vi "inverse_transform.vi"(8 "error in (no error)":errorcluster caption="entrée d'erreur (pas d'erreur)", 11 "KernelPCA.lvclass 2":refnum<class "KernelPCA.lvclass">) -> (0 "error out":errorcluster caption="sortie d'erreur", 2 "X":dbl[][](array[numeric]), 3 "KernelPCA.lvclass":refnum<class "KernelPCA.lvclass">)   [LabVIEW 2020, in "KernelPCA.lvclass"]
doc: "Transform X back to original space.\n\n ``inverse_transform`` approximates the inverse transformation using\n a learned pre-image. The pre-image is learned by kernel ridge\n regression of the original data on their low-dimensional representation\n vectors.\n\n .. note:\n :meth:`~sklearn.decomposition.fit` internally uses a centered\n kernel. As the centered kernel no longer contains the information\n of the mean of kernel features, such information is not taken into\n account in reconstruction.\n\n .. note::\n When users want to compute inverse transformation for 'linear'\n kernel, it is recommended that they use\n :class:`~sklearn.decomposition.PCA` instead. Unlike\n :class:`~sklearn.decomposition.PCA`,\n :class:`~sklearn.decomposition.KernelPCA`'s ``inverse_transform``\n does not reconstruct the mean of data when 'linear' kernel is used\n due to the use of centered kernel."
uses:
  KernelPCA.lvclass
  C:/Users/cipop/TDF Dropbox/2_Technologies de France/1 - Services et Etudes/PLAIY/2 - DEV/PLAIYLAB/code/Python/Python.lvclass
  C:/Users/cipop/TDF Dropbox/2_Technologies de France/1 - Services et Etudes/PLAIY/2 - DEV/PLAIYLAB/code/Model/Model.lvclass
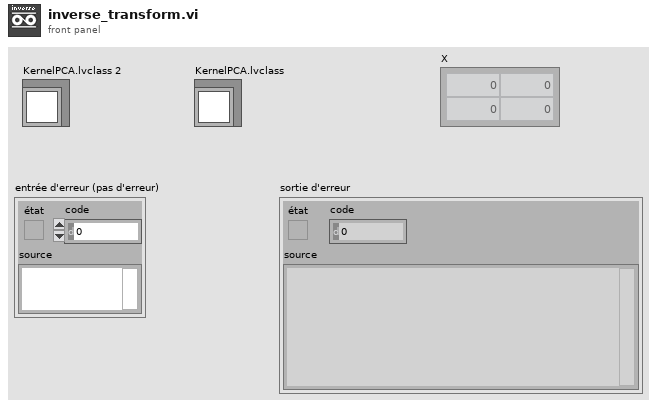
[diagram p1: front panel]
types:
  T1 = typedef "data.ctl" = cluster{"name":string, "X":dbl[][]}
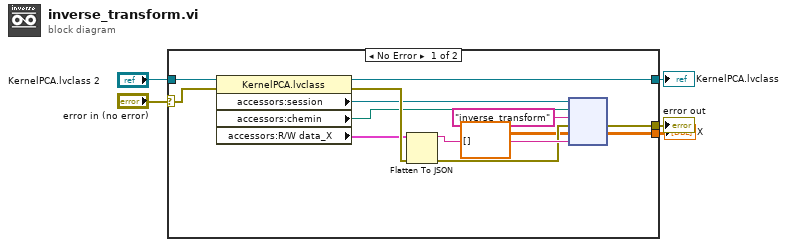
[diagram p0: block diagram]
diagram:
  n1 = case shown="No Error" "error in (no error)" {
    selector: "error in (no error)" -> [w16 w20]
    tunnel: [w17 w20] -> w4
    tunnel: [w9 w19] -> w2
    tunnel: "KernelPCA.lvclass 2" -> [w8 w19]
    tunnel: [w6 _] -> w1
    frame No Error {
      n2 = property class="KernelPCA.lvclass"(reference=w8, error in=w16) -> (reference out=w9:refnum<class "KernelPCA.lvclass">, error out=w14:errorcluster, "accessors:session"=w11:refnum<k35>, "accessors:chemin"=w10:path, "accessors:R/W data_X"=w12:T1)
      n3 = Flatten To JSON(anything=w12, error in (no error)=w14) -> (JSON string=w15:string, 11:w13:errorcluster)  [unwired: 1 in]
      n4 = node(w11, w10, "inverse_transform" ("nom de la fonction"), w13, dbl[][] [], w15) -> (w17:errorcluster, w6:dbl[][])  [unwired: 1 in, 3 out]
    }
    frame Error {
    }
  }
  "error out" <- w4
  "KernelPCA.lvclass" <- w2
  "X" <- w1
